vi "Some VI 4.vi"(8 "Error In":errorcluster) -> (0 "Error Out":errorcluster, 2 "signal out 2":waveform(dbl))   [LabVIEW 2018]
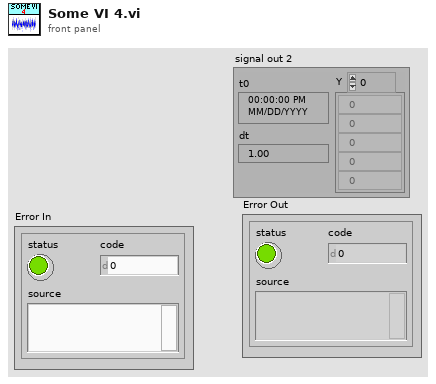
[diagram p1: front panel]
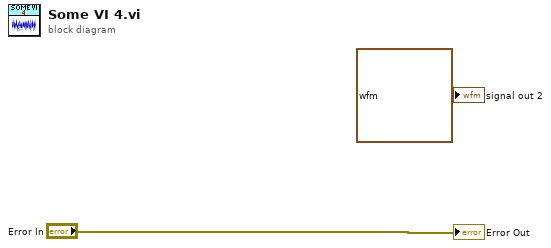
[diagram p0: block diagram]
diagram:
  "Error Out" <- "Error In"
  "signal out 2" <- waveform(dbl) {"t0"=timestamp(0 s since 1904-01-01), "dt"=1.0, "Y"=[]} ("signal out 2")
